vi "E Quit.vi"(8 "error in (no error)":errorcluster, 11 "Excel.Application":refnum<k7>) -> (0 "error out":errorcluster)   [LabVIEW 2014]
doc: "退出Excel应用程序。"
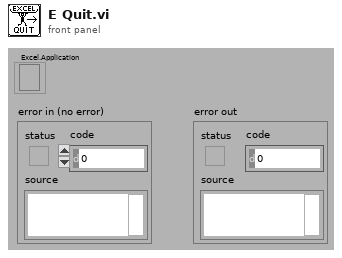
[diagram p1: front panel]
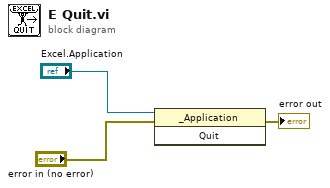
[diagram p0: block diagram]
diagram:
  n1 = invoke class="_Application" method="Quit"(reference="Excel.Application", error in="error in (no error)") -> (error out=→"error out":errorcluster)  [unwired: 1 in, 2 out]
